vi "Wait Top Level.vi"(8 "error in (no error)":errorcluster) -> (0 "error out":errorcluster)   [LabVIEW 2020, in "Wait.lvlib"]
uses:
  Wait.lvlib
  Private Controls/Module Action.ctl
  Public Controls/Module Data Cluster.ctl
  8aca9fd9-3eec-410d-ba36-3c013a116245.vi
  b2557411-5cff-4c84-9b89-16ab07a25453.vi
  27c827a8-6ce2-46ff-b742-8397f53ceddc.vi
  Controller/Controller.lvlib
  Error Handler/Error Handler.lvlib
panel:
  out "Countdown (s)":dbl
  out "Action":T1
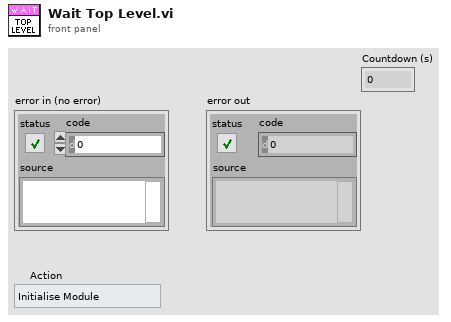
[diagram p1: front panel]
types:
  T1 = typedef "Wait.lvlib/Module Action.ctl" = enum16{"Initialise Module", "Start", "Wait", "Abort", "Error", "Exit"}
  T2 = typedef "Wait.lvlib/Module Data Cluster.ctl" = cluster{"Refresh Period":i32}
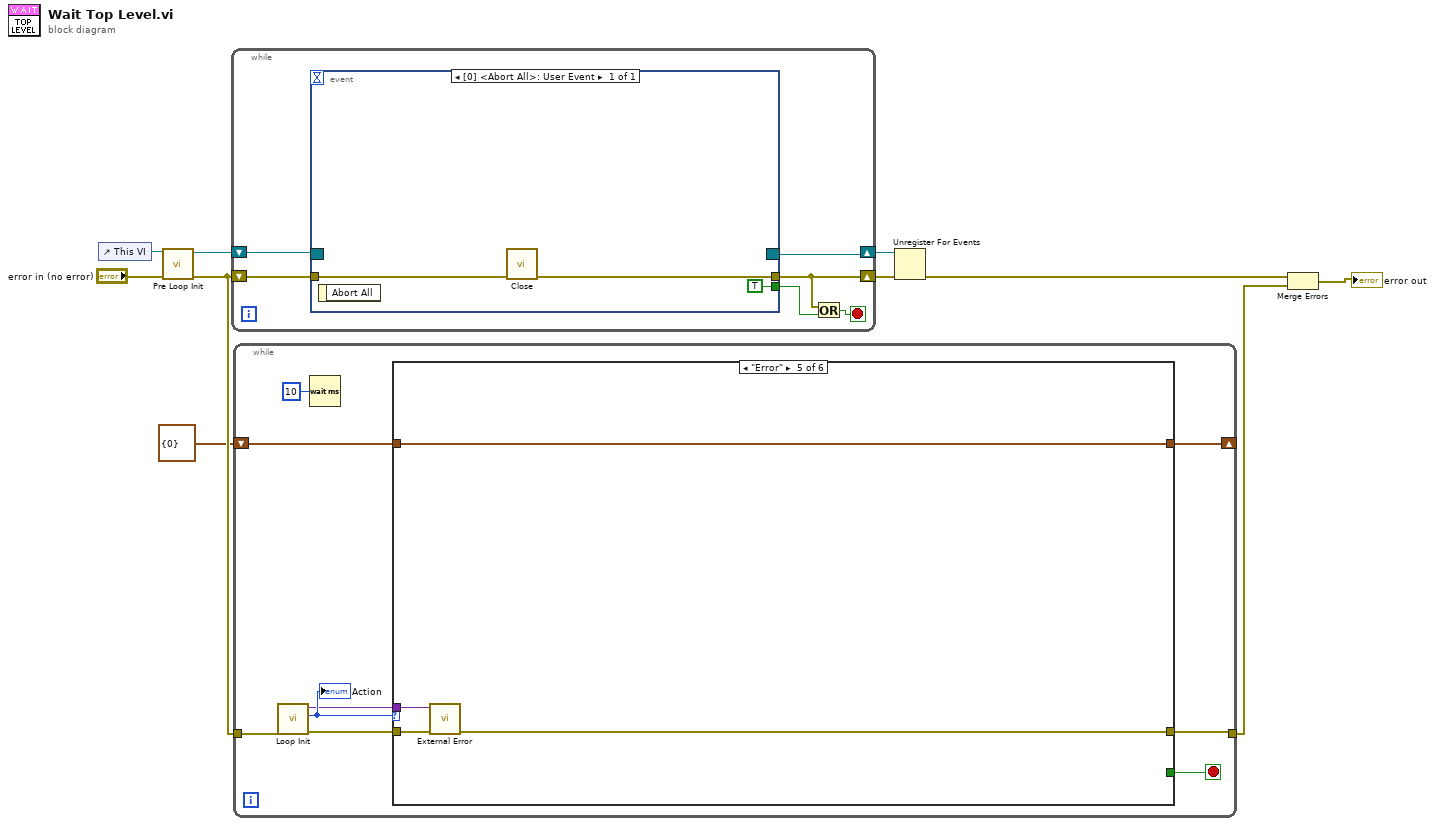
[diagram p0: block diagram]
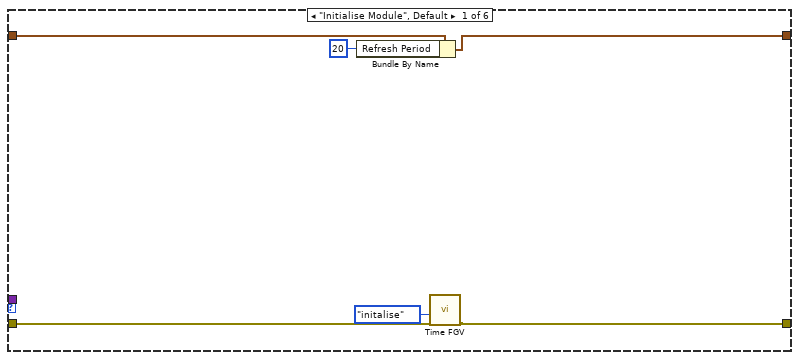
[diagram p2: hidden frame]
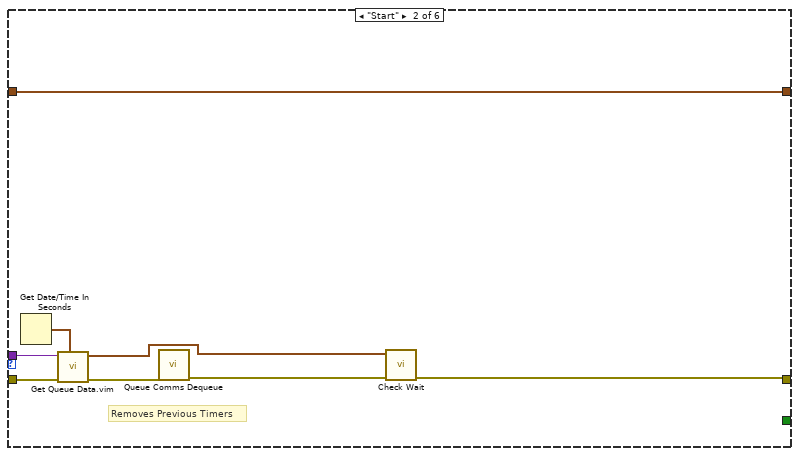
[diagram p3: hidden frame]
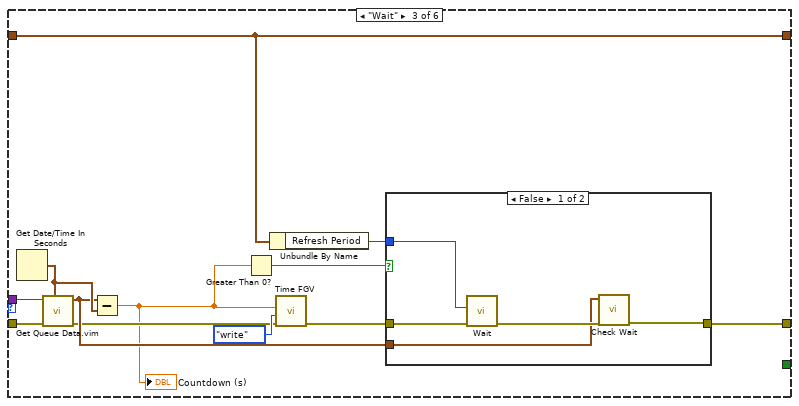
[diagram p4: hidden frame]
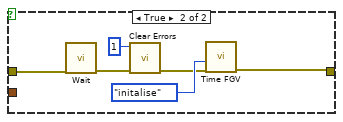
[diagram p5: hidden frame]
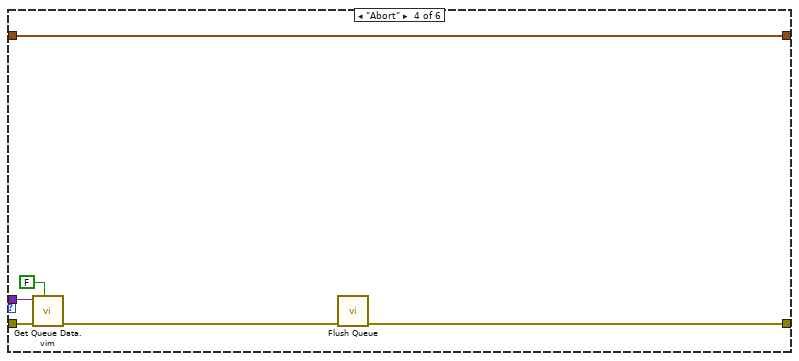
[diagram p6: hidden frame]
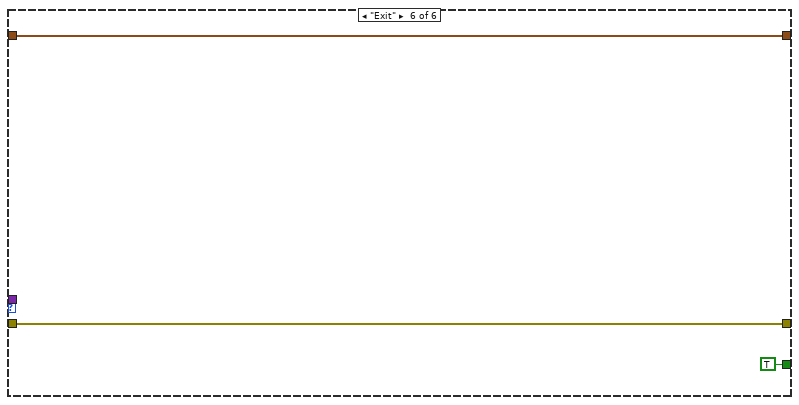
[diagram p7: hidden frame]
diagram:
  n1 = control-ref of="This VI"() -> (w3:refnum<vi>)
  n2 = call "Pre Loop Init.vi"("error in (no error)"="error in (no error)", "Ref In"=w3) -> ("error out"=w6:errorcluster, "Event Registration Refnum"=w5:refnum<event-registration>)  [unwired: 8 in]
  n3 = while {
    shift-right: [w13] -> w9
    shift-left: w6 -> [w12]
    shift-right: [w15] -> w4
    shift-left: w5 -> [w16]
    stop <- w14 stop-if-true
    n4 = event shown="[0] <Abort All>: User Event" {
      selector: w16 -> [_]
      dyn-events: [_] -> w15
      timeout: _ -> [_]
      tunnel: [w18] -> w13
      tunnel: w12 -> [w19]
      tunnel: [TRUE] -> w11
      event User Event {
        n5 = event-data() -> ()  [unwired: 1 in, 1 out]
        n6 = call "Close.vi"("error in (no error)"=w19) -> ("error out"=w18:errorcluster)  [unwired: 10 in]
      }
    }
    n7 = Or(x=w13, y=w11) -> (x .or. y?=w14:bool)
  }
  n8 = while {
    shift-right: [w22] -> _
    shift-left: T2 {"Refresh Period"=0} ("Module Data Cluster") -> [w23]
    tunnel: w6 -> [w27]
    tunnel: [w24] -> w7
    stop <- w21 stop-if-true
    n9 = call "Loop Init.vi"("error in (no error)"=w27) -> ("error out"=w25:errorcluster, "Action"=w26:T1, "Data"=w20:variant)  [unwired: 8 in]
    "Action" <- w26
    n10 = Wait (ms)(milliseconds to wait=u32 10) -> ()  [unwired: 1 out]
    n11 = case shown="\"Error\"" w26 {
      tunnel: w25 -> [w31 w41 w54 w71 w74 w76]
      tunnel: [w30 w37 w52 w66 w72 w76] -> w24
      tunnel: w23 -> [w34 w42 w49 w68 w75 w78]
      tunnel: [w33 w42 w49 w68 w75 w78] -> w22
      tunnel: [_ _ _ _ _ TRUE] -> w21
      tunnel: w20 -> [_ w40 w53 w70 w73 _]
      frame "Initialise Module", Default {
        n12 = Bundle By Name(cluster=w34, "Refresh Period"=20) -> (w33:T2)
        n13 = call "Time FGV.vi"("error in (no error)"=w31, "Enum"=enum16{"initalise", "read", "write"}."initalise") -> ("error out"=w30:errorcluster)  [unwired: 8 in, 1 out]
      }
      frame "Start" {
        # "Removes Previous Timers"
        n14 = Get Date/Time In Seconds() -> (seconds since 1Jan1904=w36:timestamp)
        n15 = call "Get Queue Data.vim"("Default Value"=w36, "error in"=w41, "Variant"=w40) -> ("error out"=w39:errorcluster, "Module Data"=w35:timestamp)  [unwired: 7 in]
        n16 = call "Queue Comms Dequeue.vi"("error in (no error)"=w39) -> ("error out"=w38:errorcluster)  [unwired: 9 in, 1 out]
        n17 = call "Check Wait.vi"("error in (no error)"=w38, "Data"=w35) -> ("error out"=w37:errorcluster)  [unwired: 9 in]
      }
      frame "Wait" {
        n18 = Get Date/Time In Seconds() -> (seconds since 1Jan1904=w51:timestamp)
        n19 = call "Get Queue Data.vim"("Default Value"=w51, "error in"=w54, "Variant"=w53) -> ("error out"=w44:errorcluster, "Module Data"=w50:timestamp)  [unwired: 7 in]
        n20 = Subtract(x=w50, y=w51) -> (x-y=w43:dbl)
        "Countdown (s)" <- w43
        n21 = Greater Than 0?(x=w43) -> (x > 0?=w47:bool)
        n22 = Unbundle By Name(w49) -> ("Refresh Period"=w48:i32)
        n23 = call "Time FGV.vi"("error in (no error)"=w44, "Enum"=enum16{"initalise", "read", "write"}."write", "Countdown (s) in"=w43) -> ("error out"=w45:errorcluster)  [unwired: 7 in, 1 out]
        n24 = case shown="False" w47 {
          tunnel: w45 -> [w59 w64]
          tunnel: [w57 w60] -> w52
          tunnel: w50 -> [w56 _]
          tunnel: w48 -> [w55 _]
          frame False {
            n25 = call "Wait.vi"("error in (no error)"=w59, "wait (0ms)"=w55) -> ("error out"=w58:errorcluster)  [unwired: 9 in]
            n26 = call "Check Wait.vi"("error in (no error)"=w58, "Data"=w56) -> ("error out"=w57:errorcluster)  [unwired: 9 in]
          }
          frame True {
            n27 = call "Wait.vi"("error in (no error)"=w64) -> ("error out"=w63:errorcluster)  [unwired: 10 in]
            n28 = call <vilib>:"Clear Errors.vi"("error in (no error)"=w63, "specific error code to clear (0: all)"=1) -> ("error out"=w61:errorcluster)  [unwired: 4 in, 1 out]
            n29 = call "Time FGV.vi"("error in (no error)"=w61, "Enum"=enum16{"initalise", "read", "write"}."initalise") -> ("error out"=w60:errorcluster)  [unwired: 8 in, 1 out]
          }
        }
      }
      frame "Abort" {
        n30 = call "Get Queue Data.vim"("Default Value"=FALSE, "error in"=w71, "Variant"=w70) -> ("error out"=w67:errorcluster)  [unwired: 7 in, 1 out]
        n31 = call "Flush Queue.vi"("error in (no error)"=w67) -> ("error out"=w66:errorcluster)  [unwired: 10 in]
      }
      frame "Error" {
        n32 = call "External Error.vi"("error in (no error)"=w74, "Data"=w73) -> ("error out"=w72:errorcluster)  [unwired: 9 in]
      }
      frame "Exit" {
      }
    }
  }
  n33 = Unregister For Events(event registration refnum=w4, error in=w9) -> (error out=w8:errorcluster)
  n34 = Merge Errors(w8, w7) -> (→"error out":errorcluster)
